vi "meth.PushVariantArray.vi"(0 "class.GLue in":refnum<class "class.GLue.lvclass">, 7 "Array":variant[](array[variant]), 11 "error in":errorcluster) -> (4 "class.GLue out":refnum<class "class.GLue.lvclass">, 8 "Pushed?":bool=TRUE, 15 "error out":errorcluster)   [LabVIEW 2014, in "GLue.lvlib" / "class.GLue.lvclass"]
uses:
  class.GLue.lvclass
  class.GLue.lvclass/class.GLue.ctl
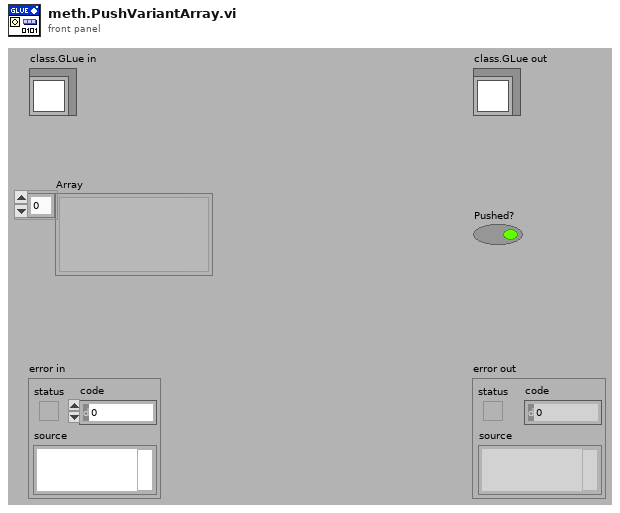
[diagram p1: front panel]
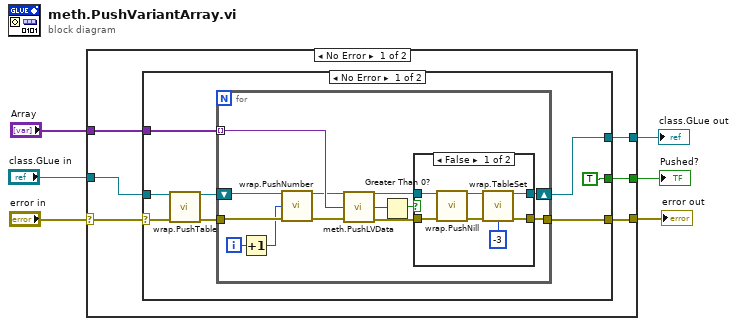
[diagram p0: block diagram]
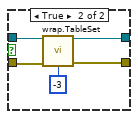
[diagram p2: hidden frame]
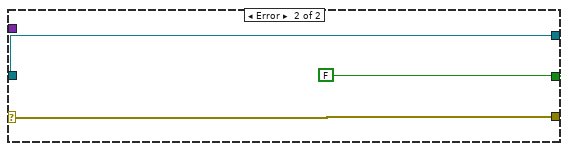
[diagram p4: hidden frame]
diagram:
  n1 = case shown="No Error" "error in" {
    selector: "error in" -> [w7 w51]
    tunnel: [w12 w51] -> w6
    tunnel: [w10 w50] -> w4
    tunnel: "class.GLue in" -> [w11 w50]
    tunnel: [w9 FALSE] -> w2
    tunnel: "Array" -> [w8 _]
    frame No Error {
      n2 = case shown="No Error" w7 {
        selector: w7 -> [w18 w48]
        tunnel: w8 -> [w20 _]
        tunnel: [w14 w48] -> w12
        tunnel: w11 -> [w16 w47]
        tunnel: [w19 w47] -> w10
        tunnel: [TRUE FALSE] -> w9
        frame No Error {
          n3 = call "wrap.PushTable.vi"("class.GLue in"=w16, "error in (no error)"=w18) -> ("class.GLue out"=w15:refnum<class "class.GLue.lvclass">, "error out"=w17:errorcluster)  [unwired: 12 in]
          n4 = for {
            tunnel: w20 -> [w33] mode=indexing
            tunnel: w17 -> [w25]
            shift-right: [w28] -> w19
            shift-left: w15 -> [w24]
            tunnel: [w27] -> w14
            i -> [w22]
            stop <- w27 stop-if-true
            n5 = Increment(x=w22) -> (x+1=w21:i32)
            n6 = call "wrap.PushNumber.vi"("class.GLue in"=w24, "Numeric"=w21, "error in (no error)"=w25) -> ("class.GLue out"=w23:refnum<class "class.GLue.lvclass">, "error out"=w26:errorcluster)  [unwired: 11 in]
            n7 = call "meth.PushLVData.vi"("class.GLue in"=w23, "variant in"=w33, "error in (no error)"=w26) -> ("class.GLue out"=w30:refnum<class "class.GLue.lvclass">, "NumPushed"=w32:i32, "error out"=w29:errorcluster)  [unwired: 10 in]
            n8 = Greater Than 0?(x=w32) -> (x > 0?=w31:bool)
            n9 = case shown="False" w31 {
              tunnel: w30 -> [w40 w44]
              tunnel: w29 -> [w39 w45]
              tunnel: [w35 w41] -> w27
              tunnel: [w34 w42] -> w28
              frame False {
                n10 = call "wrap.PushNill.vi"("class.GLue in"=w40, "error in (no error)"=w39) -> ("class.GLue out"=w36:refnum<class "class.GLue.lvclass">, "error out"=w37:errorcluster)  [unwired: 12 in]
                n11 = call "wrap.TableSet.vi"("class.GLue in"=w36, "error in (no error)"=w37, "Index"=-3) -> ("class.GLue out"=w34:refnum<class "class.GLue.lvclass">, "error out"=w35:errorcluster)  [unwired: 11 in]
              }
              frame True {
                n12 = call "wrap.TableSet.vi"("class.GLue in"=w44, "error in (no error)"=w45, "Index"=-3) -> ("class.GLue out"=w42:refnum<class "class.GLue.lvclass">, "error out"=w41:errorcluster)  [unwired: 11 in]
              }
            }
          }
        }
        frame Error {
        }
      }
    }
    frame Error {
    }
  }
  "error out" <- w6
  "class.GLue out" <- w4
  "Pushed?" <- w2
